vi "Config.vi"(11 "Module in":refnum<class "Module.lvclass">) -> (2 "Config":refnum<class "VolatusConfigElement.lvclass">, 3 "Module out":refnum<class "Module.lvclass">)   [LabVIEW 2020, in "Volatus.lvlib" / "Module.lvclass"]
uses:
  Module.lvclass
  VolatusConfig/VolatusConfigElement/VolatusConfigElement.lvclass
  Module.lvclass/Module.ctl
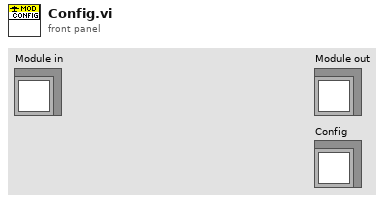
[diagram p1: front panel]
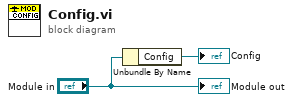
[diagram p0: block diagram]
diagram:
  n1 = Unbundle By Name("Module in") -> ("Config"=→"Config":refnum<class "VolatusConfigElement.lvclass">)
  "Module out" <- "Module in"
